vi "Utility - extract ROI from critta tracking settings.vi"() -> ()   [LabVIEW 2013]
uses:
  <vilib>/Utility/file.llb/Write To Spreadsheet File (I64).vi
panel:
  out "ROI rectangle":i32[][](array[numeric])
  in  "transpose":bool=TRUE
  in  "tracking settings file":path
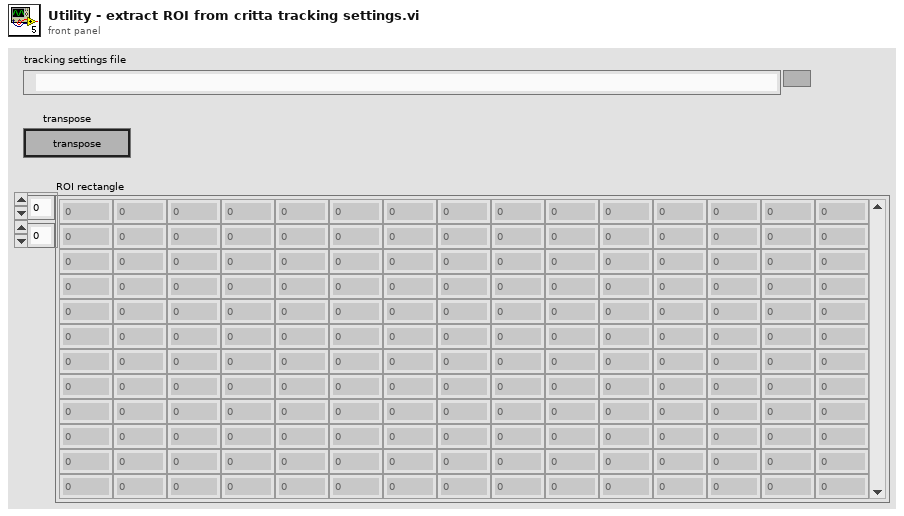
[diagram p1: front panel]
types:
  T1 = cluster{"ROI":cluster{"ID":string, "Enabled":bool, "Process settings":cluster{"Light object":bool, "Threshold":sgl, "Open enabled":bool, "Open value":i32, "Close enabled":bool, "Close value":i32, "Fill enabled":bool, "min area":i32, "max area":i32}, "ROI rectangle":cluster{"left":i32, "top":i32, "right":i32, "bottom":i32}, "Calc params":cluster{"ROI % X scale":sgl, "ROI % Y scale":sgl, "ROI width":sgl, "ROI height":sgl, "ROI center X":sgl, "ROI center Y":sgl}, "Profile settings":cluster{"Threshold":sgl, "Object width":i32, "Orientation":enum16{"X", "Y", "X & Y"}}, "BG method":enum16{"None", "Min/Max hold", "Outline mask", "Square mask"}}[], "ROI shape":enum32{"Rectangular", "Circular"}, "#rows":i32, "#columns":i32, "Cmn calc params":cluster{"scale":cluster{"X mm/pix":sgl, "Y mm/pix":sgl}, "Velocity Averaging":cluster{"Averaging mode":enum16{"Weighted Moving Average", "Exponential Moving Average"}, "EMA coefficient":sgl, "Weights":sgl[], "Rebound filter":bool}}, "Ref ROI":cluster{"Ref threshold":i32, "ROIs":cluster{"left":i32, "top":i32, "right":i32, "bottom":i32}[], "Stable count":i32}, "Method":enum16{"Silhouette (X & Y)", "Profile (X only)", "Motion detection"}, "Colour conversion":enum16{"None", "Convert colour to greyscale", "Use only Red plane", "Use only Green plane", "Use only Blue plane"}}
  T2 = cluster{"ID":string, "Enabled":bool, "Process settings":cluster{"Light object":bool, "Threshold":sgl, "Open enabled":bool, "Open value":i32, "Close enabled":bool, "Close value":i32, "Fill enabled":bool, "min area":i32, "max area":i32}, "ROI rectangle":cluster{"left":i32, "top":i32, "right":i32, "bottom":i32}, "Calc params":cluster{"ROI % X scale":sgl, "ROI % Y scale":sgl, "ROI width":sgl, "ROI height":sgl, "ROI center X":sgl, "ROI center Y":sgl}, "Profile settings":cluster{"Threshold":sgl, "Object width":i32, "Orientation":enum16{"X", "Y", "X & Y"}}, "BG method":enum16{"None", "Min/Max hold", "Outline mask", "Square mask"}}[]
  T3 = cluster{"left":i32, "top":i32, "right":i32, "bottom":i32}
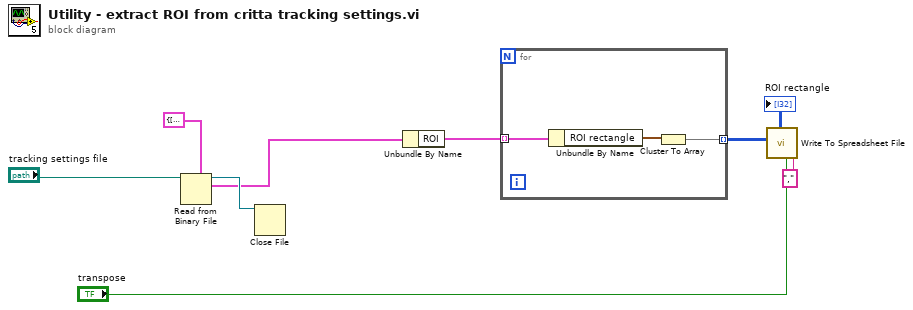
[diagram p0: block diagram]
diagram:
  n1 = Read from Binary File(5:T1 {"ROI"=[], "ROI shape"=enum."Rectangular", "#rows"=1, "#columns"=1, "Cmn calc params"={"scale"={"X mm/pix"=0.0, "Y mm/pix"=0.0}, "Velocity Averaging"={"Averaging mode"=enum."Weighted Moving Average", "EMA coefficient"=0.0, "Weights"=[], "Rebound filter"=FALSE}}, "Ref ROI"={"Ref threshold"=0, "ROIs"=[], "Stable count"=0}, "Method"=enum."Silhouette (X & Y)", "Colour conversion"=enum."None"} ("Tracker settings"), 11:"tracking settings file") -> (2:w5:T1, 3:w6:refnum<file>)  [unwired: 4 in, 2 out]
  n2 = Close File(refnum=w6) -> ()  [unwired: 1 in, 2 out]
  n3 = Unbundle By Name(w5) -> ("ROI"=w4:T2)
  n4 = for {
    tunnel: w4 -> [w11] mode=indexing
    tunnel: [w9] -> w3 mode=indexing
    n5 = Unbundle By Name(w11) -> ("ROI rectangle"=w10:T3)
    n6 = Cluster To Array(cluster=w10) -> (array=w9:i32[])
  }
  "ROI rectangle" <- w3
  n7 = call-poly <vilib>:"Write To Spreadsheet File.vi"("delimiter (\\t)"="," ("delimiter (\\t)"), "transpose? (no:F)"="transpose", "2D data"=w3) -> ()  [unwired: 5 in, 1 out]
